vi "Offset Inline Buffer.vi"(8 "error in (no error)":errorcluster, 9 "group engine offset":u64, 10 "Engine Pointer":refnum<class "Memory.Pointer.lvclass">, 11 "Transfer in":refnum<class "Transfer.lvclass">) -> (0 "error out":errorcluster, 3 "Transfer out":refnum<class "Transfer.lvclass">)   [LabVIEW 2017, in "Data Sharing Framework Core.lvlib" / "Data Sharing Framework Engine.lvlib" / "Transfer.lvclass"]
uses:
  Transfer.lvclass
  <vilib>/National Instruments/Memory Manager/Classes/Pointer/Memory.Pointer.lvclass
  Transfer.lvclass/Transfer.ctl
  Internal/Memory/Double Pointer/Double Pointer.lvclass
  C:/Program Files (x86)/National Instruments/LabVIEW 2017/vi.lib/National Instruments/Memory Manager/Classes/Pointer/Memory.Pointer.lvclass
  <vilib>/National Instruments/Memory Manager/Classes/Pointer/Memory.Pointer.lvclass/Memory.Pointer.ctl
  <vilib>/National Instruments/Memory Manager/Classes/Pointer/Memory.Pointer.Parameter Check.Subset.vi
  <vilib>/National Instruments/Memory Manager/Classes/Pointer/Memory.Pointer.Get Address.vi
  <vilib>/National Instruments/Memory Manager/Classes/Pointer/Memory.Pointer.Encapsulate.vi
  <vilib>/National Instruments/Memory Manager/Classes/Pointer/Memory.Pointer.Parameter Check.Null Pointer.vi
  <vilib>/National Instruments/Memory Manager/Classes/Pointer/Memory.Pointer.Errors.vi
  <vilib>/National Instruments/Memory Manager/Classes/Pointer/Memory.Pointer.Errors.Out of Bounds.vi
  <vilib>/National Instruments/Memory Manager/Classes/Pointer/Memory.Pointer.Get Size.vi
  <vilib>/National Instruments/Memory Manager/Classes/Pointer/Memory.Pointer.Set Size.vi
  <vilib>/National Instruments/Memory Manager/Classes/Pointer/Memory.Pointer.Set Address.vi
  <vilib>/National Instruments/Memory Manager/Classes/Pointer/Memory.Pointer.Set Allocated.vi
  <vilib>/National Instruments/Memory Manager/Classes/Pointer/Memory.Pointer.Errors.Null Pointer.vi
  <vilib>/NI/Static Error Handling/VIs/Static Error Handling.Source Buffer.Write.String.vi
  <vilib>/National Instruments/Memory Manager/Classes/Pointer/Memory.Pointer.Errors.Write Pointer Size.vi
  <vilib>/National Instruments/Memory Manager/Classes/Pointer/Memory.Pointer.Errors.Create Error.vi
  <vilib>/NI/Static Error Handling/VIs/Static Error Handling.Source Buffer.Write.Numeric.Scalar.Base10.vi
  <vilib>/NI/Static Error Handling/VIs/Static Error Handling.Source Buffer.Write.Numeric.Scalar.Base10 (U64).vi
  <vilib>/NI/Static Error Handling/VIs/Static Error Handling.Error Cluster Constant.vi
  <vilib>/NI/Static Error Handling/VIs/Static Error Handling.Error Cluster Constant (512B).vi
  <vilib>/NI/Static Error Handling/VIs/Static Error Handling.Parameters.Status.Set.vi
  <vilib>/NI/Static Error Handling/VIs/Static Error Handling.Parameters.Code.Set.vi
  <vilib>/NI/Static Error Handling/VIs/Static Error Handling.Parameters.VI Source.Set.vi
  <vilib>/National Instruments/Memory Manager/Constants/Memory.Constants.vi
  <vilib>/National Instruments/Memory Manager/Constants/Memory.Constants.Library Name.vi
  <vilib>/National Instruments/Memory Manager/Classes/Pointer/Memory.Pointer.Errors.Get Info.vi
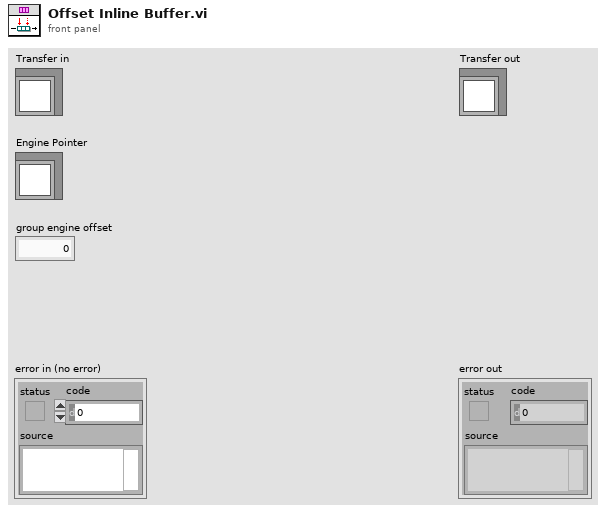
[diagram p1: front panel]
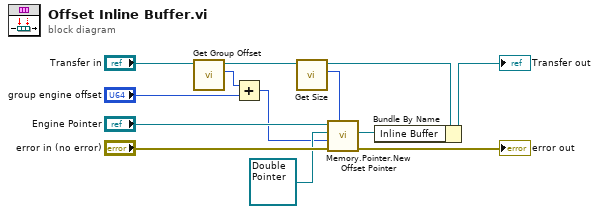
[diagram p0: block diagram]
diagram:
  n1 = call "Get Group Offset.vi"("Transfer in"="Transfer in") -> ("group offset"=w9:u64, "Transfer out"=w7:refnum<class "Transfer.lvclass">)  [unwired: 9 in]
  n2 = Add(x=w9, y="group engine offset") -> (x+y=w1:u64)
  n3 = call "Get Size.vi"("Transfer in"=w7) -> ("size"=w2:u64, "Transfer out"=w6:refnum<class "Transfer.lvclass">)  [unwired: 9 in]
  n4 = call <vilib>:"Memory.Pointer.New Offset Pointer.vi"("length (-1: rest)"=w2, "error in (no error)"="error in (no error)", "offset (0)"=w1, "offset Pointer type"=refnum<class "Double Pointer.lvclass"> refnum ("Inline Buffer"), "base Pointer in"="Engine Pointer") -> ("error out"=→"error out":errorcluster, "offset Pointer"=w3:refnum<class "Double Pointer.lvclass">)  [unwired: 3 in, 2 out]
  n5 = Bundle By Name(cluster=w6, "Inline Buffer"=w3) -> (→"Transfer out":refnum<class "Transfer.lvclass">)
